vi "Read Behavior.vi"(11 "Filter in":refnum<class "Filter.lvclass">) -> (2 "match behavior":T1, 3 "Filter out":refnum<class "Filter.lvclass">)   [LabVIEW 2024, in "Logging.lvlib" / "Filter.lvclass"]
uses:
  Filter.lvclass
  Filter.lvclass/Filter.ctl
  Match Behavior.ctl
  Logging.lvlib
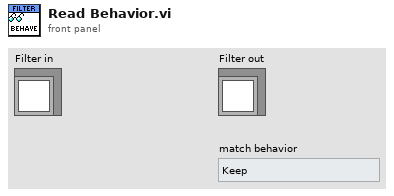
[diagram p1: front panel]
types:
  T1 = typedef "Logging.lvlib/Match Behavior.ctl" = enum16{"Keep", "Discard"}
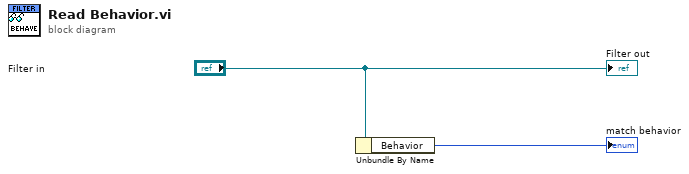
[diagram p0: block diagram]
diagram:
  n1 = Unbundle By Name("Filter in") -> ("Behavior"=→"match behavior":T1)
  "Filter out" <- "Filter in"
